vi "resonant.scan.engine.8or12kHz5ch_MD.vi"() -> ()   [LabVIEW 2012]
uses:
  <vilib>/Utility/VariantDataType/Type.ctl
  GFG/GFGbooleanGet.vi
  GFG/GFGnumericGet.vi
  GFG/GFGfpRefGet.vi
  <vilib>/Utility/error.llb/Error Cluster From Error Code.vi
  <vilib>/RVI Host/nirviSupport.llb/nirviErrorClusterFromErrorCode.vi
  <vilib>/rvi/errors/niLvFpgaAdjustHostInterfaceError.vi
  <vilib>/FPGAPlugInAG/PXIe-7962R/niLvFpga_Abort_PXIe-7962R.vi
  <vilib>/FPGAPlugInAG/PXIe-7962R/niLvFpga_Close_PXIe-7962R.vi
  <vilib>/rvi/interface/nirviMethod/nirviMethod.xnode
  FPGA/FPGA lvproj/FPGA Bitfiles/4chresonancescan_PXIe-7962R_5ch8or12kHzreson_D7lwWdudtb8.lvbitx
  <vilib>/rvi/interface/nirviCloseFPGA/nirviCloseFPGA.xnode
  GFG/GFG library.lvlib
  <vilib>/Utility/VariantDataType/VariantType.lvlib
  <vilib>/rvi/errors/niLvFpgaMergeErrorWithErrorCode.vi
  <vilib>/rvi/interface/nirviMethod/StockFPGA_InlinedMethodWaitForSingleIRQ.vi
  <vilib>/FPGAPlugInAG/PXIe-7962R/niLvFpga_WaitOnIrq_PXIe-7962R.vi
  <vilib>/FPGAPlugInAG/PXIe-7962R/niLvFpga_AcknowledgeIrq_PXIe-7962R.vi
  <vilib>/FPGAPlugInAG/PXIe-7962R/niLvFpga_ReadFifo_PXIe-7962R.vi
panel:
  out "x/y":dbl format="%#_6f"
  out "max Elements Remaining 2":u32
  out "Array":i16[][][](array[numeric])
  out "size(s)":i32[](array[numeric])
  out "Elements Remaining":u32
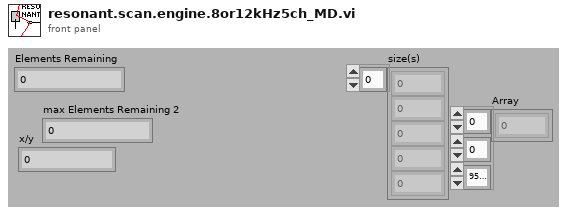
[diagram p1: front panel]
types:
  T1 = enum8{"Enabled", "Disabled", "Disabled and Grayed Out"}
  T2 = cluster{"WaveformChartRef":refnum<vi>, "DigitalRef":refnum<vi>, "ArrayRef":refnum<vi>, "TabControlRef":refnum<vi>, "EnumRef":refnum<vi>, "RingRef":refnum<vi>, "BooleanRef":refnum<vi>, "KnobRef":refnum<vi>, "SlideRef":refnum<vi>, "PathRef":refnum<vi>, "StringRef":refnum<vi>, "ComboBox":refnum<vi>, "WaveformGraphRef":refnum<vi>}
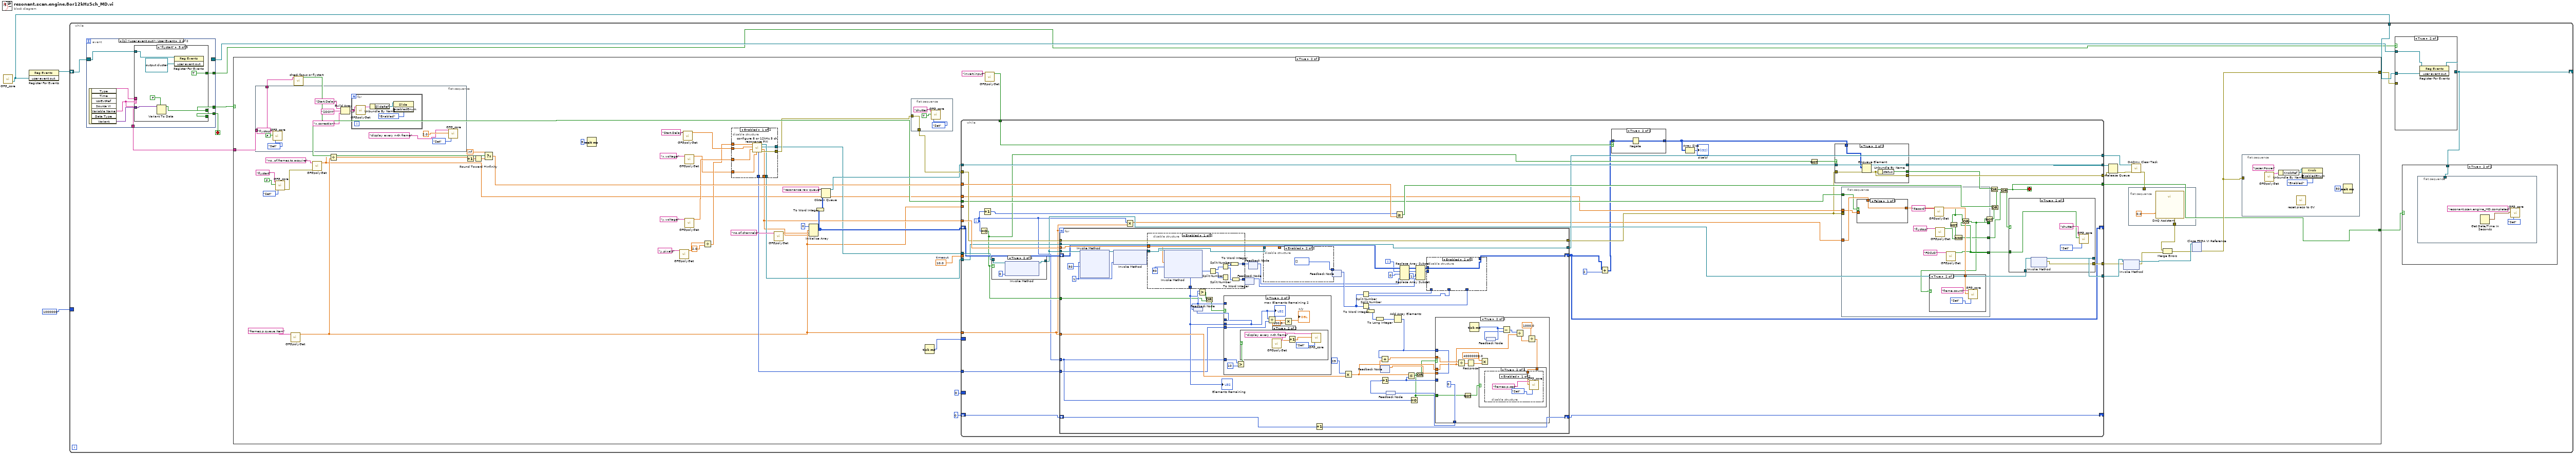
[diagram p0: block diagram]
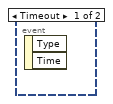
[diagram p4: hidden frame]
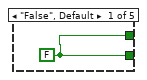
[diagram p5: hidden frame]
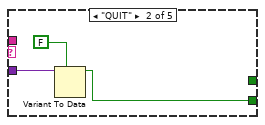
[diagram p6: hidden frame]
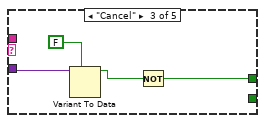
[diagram p7: hidden frame]
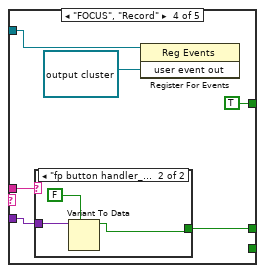
[diagram p8: hidden frame]
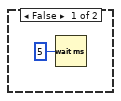
[diagram p10: hidden frame]
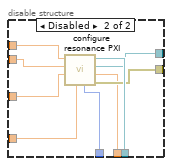
[diagram p11: hidden frame]
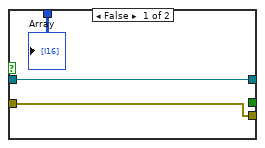
[diagram p12: hidden frame]
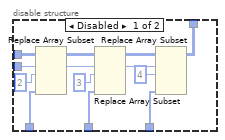
[diagram p13: hidden frame]
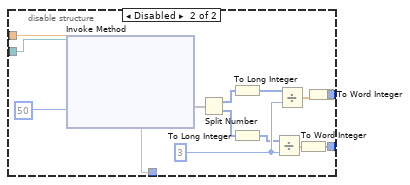
[diagram p14: hidden frame]
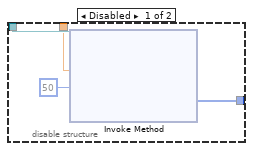
[diagram p15: hidden frame]
diagram:
  n1 = call "GFG_core.vi"() -> ("user event out"=w2:refnum<user-event>)  [unwired: 13 in, 6 out]
  n2 = register-events(w2) -> (reference out=w3:refnum<event-registration>)  [unwired: 2 in, 1 out]
  n3 = while {
    shift-right: [w4] -> _
    shift-left: w3 -> [w11]
    tunnel: w2 -> [w10]
    border: u32 1000000 ("Elements Remaining") -> [_]
    stop <- w12 stop-if-true
    n4 = event shown="[1] <user event out>: User Event" {
      selector: w11 -> [_ w24]
      dyn-events: [_ _] -> w8
      timeout: _ -> [_ _]
      tunnel: [_ w28] -> w13
      tunnel: [_ w27] -> w12
      tunnel: [_ w23] -> w7
      tunnel: [_ w22] -> w6
      event Timeout {
        n5 = event-data() -> ()  [unwired: 1 in, 2 out]
      }
      event User Event {
        n6 = event-data() -> ("Source VI"=w25:string, "Variable Name"=w22:string, "Variant"=w26:variant)  [unwired: 1 in, 4 out]
        n7 = case shown="\"flystart\"" w22 {
          tunnel: [w29 _ w33 w41 w46] -> w28
          tunnel: [w29 w30 _ _ _] -> w27
          tunnel: w26 -> [_ w32 w35 w42 w50]
          tunnel: w25 -> [_ _ _ w40 _]
          tunnel: w24 -> [_ _ _ w38 w47]
          tunnel: [_ _ _ TRUE TRUE] -> w23
          frame "False", Default {
            w29 = FALSE ("NewVal")
          }
          frame "QUIT" {
            n8 = Variant To Data(type=FALSE ("NewVal"), Variant=w32) -> (data=w30:bool)  [unwired: 1 in, 1 out]
          }
          frame "Cancel" {
            n9 = Variant To Data(type=FALSE ("NewVal"), Variant=w35) -> (data=w34:bool)  [unwired: 1 in, 1 out]
            n10 = Not(x=w34) -> (.not. x?=w33:bool)
          }
          frame "FOCUS", "Record" {
            n11 = case shown="\"fp button handler_MD.vi\"" w40 {
              tunnel: w42 -> [_ w44]
              tunnel: [_ w43] -> w41
              frame "False", Default {
              }
              frame "fp button handler_MD.vi" {
                n12 = Variant To Data(type=FALSE ("NewVal"), Variant=w44) -> (data=w43:bool)  [unwired: 1 in, 1 out]
              }
            }
            n13 = register-events(reference=w38, refnum<user-event> refnum ("user event out")) -> ()  [unwired: 1 in, 2 out]
          }
          frame "flystart" {
            n14 = Variant To Data(type=FALSE ("NewVal"), Variant=w50) -> (data=w46:bool)  [unwired: 1 in, 1 out]
            n15 = register-events(reference=w47, refnum<user-event> refnum ("user event out")) -> ()  [unwired: 1 in, 2 out]
          }
        }
      }
    }
    n16 = case shown="True" w13 {
      tunnel: [_ w88] -> w9
      tunnel: w6 -> [_ w56]
      tunnel: [_ w78] -> w5
      frame False {
        n17 = Wait (ms)(milliseconds to wait=u32 5) -> ()  [unwired: 1 out]
      }
      frame True {
        w109 = 10.0  # timeout
        n18 = flat-sequence {
          tunnel: w56 -> [w138]
          tunnel: [w138] -> w55
          frame #0 {
            n19 = call "GFG_core.vi"("Variable Name in"="flystop", "Variant in"=FALSE ("Boolean"), "Action"=enum16{"Init", "Set", "Get"}."Set") -> ()  [unwired: 10 in, 7 out]
            n20 = Build Array("Start.Delay" ("Variable Name in"), "ZOOM" ("Variable Name in"), "x.correction" ("Variable Name in")) -> (w133:string[])
            n21 = for {
              tunnel: w133 -> [w141] mode=indexing
              n22 = call-poly "GFGpolyGet.vi"("Variable Name in"=w141) -> ("output cluster"=w144:T2)  [unwired: 9 in, 1 out]
              n23 = Unbundle By Name(w144) -> ("SlideRef"=w142:refnum<vi>)
              n24 = property class="Slide"(reference=w142, "DisabledEnum"=T1."Enabled" ("Disabled")) -> ()  [unwired: 1 in, 2 out]
            }
            n25 = call "GFG_core.vi"("Variable Name in"="display every n-th frame" ("Tag in"), "Variant in"=2.0 ("Numeric"), "Action"=enum16{"Init", "Set", "Get"}."Set") -> ()  [unwired: 10 in, 7 out]
          }
        }
        n26 = call "GFG_core.vi"("Variable Name in"="flystart" ("Tag in"), "Variant in"=FALSE, "Action"=enum16{"Init", "Set", "Get"}."Set") -> ("error out"=w79:errorcluster)  [unwired: 10 in, 6 out]
        n27 = call-poly "GFGpolyGet.vi"("Variable Name in"="frames.p.queue.item" ("Tag in")) -> ("Numeric"=w61:dbl)  [unwired: 9 in, 1 out]
        n28 = call "check focus or flystart.vi"("x"=w55) -> ("x .or. y?"=w84:bool)  [unwired: 10 in]
        n29 = call-poly "GFGpolyGet.vi"("error in (no error)"=w79, "Variable Name in"="no..of.frames.to.acquire" ("Tag in")) -> ("Numeric"=w60:dbl)  [unwired: 8 in, 1 out]
        n30 = Divide(x=w60, y=w61) -> (x/y=w62:dbl)
        n31 = Increment(x=w62) -> (x+1=w57:dbl)
        n32 = Round Toward +Infinity(x=w57) -> (ceil(x): smallest int >= x=w59:dbl)
        n33 = Select(t=inf, s=w84, f=w59) -> (s? t:f=w85:dbl)
        n34 = Wait (ms)(milliseconds to wait=u32 5) -> ()  [unwired: 1 out]
        n35 = call-poly "GFGpolyGet.vi"("Variable Name in"="y.pixels" ("Tag in")) -> ("Numeric"=w103:dbl)  [unwired: 9 in, 1 out]
        n36 = call-poly "GFGpolyGet.vi"("Variable Name in"="Start.Delay" ("Tag in")) -> ("Numeric"=w75:dbl)  [unwired: 9 in, 1 out]
        n37 = call-poly "GFGpolyGet.vi"("Variable Name in"="x.voltage" ("Tag in")) -> ("Numeric"=w72:dbl)  [unwired: 9 in, 1 out]
        n38 = call-poly "GFGpolyGet.vi"("Variable Name in"="y.voltage" ("Tag in")) -> ("Numeric"=w74:dbl)  [unwired: 9 in, 1 out]
        n39 = Divide(x=w103, y=2.0 ("x")) -> (x/y=w73:dbl)
        n40 = disable-structure shown="Enabled" {
          disable-tunnel: w75 -> [w120 w123]
          disable-tunnel: w74 -> [w119 w125]
          disable-tunnel: w73 -> [w118 w122]
          disable-tunnel: w72 -> [w117 w124]
          disable-tunnel: [w116 w127] -> w71
          disable-tunnel: [w115 w129] -> w70
          disable-tunnel: [w114 w126] -> w66
          disable-tunnel: [w112 w128] -> w65
          disable-tunnel: [w113 w121] -> w63
          frame Enabled {
            n41 = call "configure 8 or 12kHz 5 ch resonance PXI.vi"("x resonant zoom voltage"=w117, "y-voltage"=w119, "Start Delay (Ticks)"=w120, "lines (2pi) per frame"=w118) -> ("error out"=w116:errorcluster, "pixels per frame"=w114:dbl, "FPGA VI Reference Out"=w112:refnum<k20>, "AO task out"=w115:refnum<k21>, "Actual Depth 3"=w113:u32)  [unwired: 3 in]
          }
          frame Disabled {
            n42 = call "configure resonance PXI.vi"("x resonant zoom voltage"=w124, "y-voltage"=w125, "Start Delay (Ticks)"=w123, "lines (2pi) per frame"=w122) -> ("error out"=w127:errorcluster, "pixels per frame"=w126:dbl, "FPGA VI Reference Out"=w128:refnum<k20>, "AO task out"=w129:refnum<k21>, "Actual Depth"=w121:u32)  [unwired: 3 in]
          }
        }
        n43 = call-poly "GFGpolyGet.vi"("Variable Name in"="no.of.channels" ("Tag in")) -> ("Numeric"=w69:dbl)  [unwired: 9 in, 1 out]
        n44 = Initialize Array(i16 0, w61, w69, w66) -> (w95:i16[][][])
        n45 = To Word Integer(number=w95) -> (16bit integer=w53:i16[][][])
        n46 = Obtain Queue(name (unnamed)="resonance raw queue", element data type=w53) -> (queue out=w96:refnum<queue>)  [unwired: 3 in, 2 out]
        n47 = flat-sequence {
          tunnel: [w152] -> w105
          tunnel: w71 -> [w152]
          frame #0 {
            n48 = call "GFG_core.vi"("Variable Name in"="shutter" ("Tag in"), "Variant in"=TRUE, "Action"=enum16{"Init", "Set", "Get"}."Set") -> ()  [unwired: 10 in, 7 out]
          }
        }
        n49 = Tick Count (ms)() -> (millisecond timer value=w54:u32)
        n50 = call-poly "GFGpolyGet.vi"("Variable Name in"="invert.input" ("Tag in")) -> ("Boolean"=w106:bool)  [unwired: 10 in]
        n51 = while {
          tunnel: w70 -> [w182]
          tunnel: [w181] -> w111
          tunnel: [w192] -> w68
          tunnel: w96 -> [w195]
          tunnel: [w194] -> w110
          tunnel: w85 -> [w193]
          tunnel: w109 -> [_]
          tunnel: w105 -> [w183]
          tunnel: w106 -> [w190]
          tunnel: w65 -> [w186]
          tunnel: w66 -> [w184]
          tunnel: [w180] -> w94
          tunnel: [w179] -> w92
          tunnel: w84 -> [w178]
          tunnel: w60 -> [w177]
          tunnel: [w172] -> w78
          shift-right: [w158] -> _
          shift-left: w95 -> [w185]
          tunnel: w61 -> [w164]
          tunnel: w61 -> [_]
          border: 0 ("x+y") -> [_]
          tunnel: w63 -> [w166]
          shift-right: [w161] -> _
          shift-left: 0 ("x+y") -> [w162]
          border: w54 -> [_]
          i -> [w160]
          stop <- w172 stop-if-true
          n52 = Equal To 0?(x=w160) -> (x = 0?=w167:bool)
          n53 = Increment(x=w160) -> (x+1=w163:i32)
          n54 = case shown="True" w167 {
            tunnel: w186 -> [w331 w334]
            tunnel: [w331 w333] -> w171
            frame False {
            }
            frame True {
              n55 = xnode "Invoke Method"("FPGA VI Reference In"=w334, "IRQ Number(s)"=0) -> ("FPGA VI Reference Out"=w333:refnum<k20>)  [unwired: 1 in, 1 out]
            }
          }
          n56 = for {
            N: w164 -> [_]
            tunnel: [w254] -> w168
            tunnel: w183 -> [w254]
            tunnel: w182 -> [w252]
            tunnel: w184 -> [w250]
            tunnel: w171 -> [w253]
            shift-right: [w244] -> w158
            shift-left: w185 -> [w248]
            tunnel: [w252] -> w181
            tunnel: w164 -> [w232]
            tunnel: w167 -> [w224]
            tunnel: w166 -> [w223]
            shift-right: [w221] -> w161
            shift-left: w162 -> [w222]
            tunnel: w160 -> [w214]
            i -> [w243]
            w220 = 1 ("IRQ Number(s)")
            n57 = xnode "Invoke Method"("FPGA VI Reference In"=w253, "IRQ Number(s)"=w220, "Timeout (ms)"=50) -> ("FPGA VI Reference Out"=w219:refnum<k20>)  [unwired: 1 in, 3 out]
            n58 = xnode "Invoke Method"("FPGA VI Reference In"=w219, "IRQ Number(s)"=w220) -> ("FPGA VI Reference Out"=w251:refnum<k20>)  [unwired: 1 in, 1 out]
            n59 = disable-structure shown="Enabled" {
              disable-tunnel: w251 -> [w277 w287]
              disable-tunnel: w250 -> [w276 w286]
              disable-tunnel: [w275 w280] -> w228
              disable-tunnel: [w268 w282] -> w208
              disable-tunnel: [w267 w281] -> w207
              frame Enabled {
                n60 = xnode "Invoke Method"("FPGA VI Reference In"=w277, "Number of Elements"=w276, "Timeout (ms)"=50) -> ("Data"=w273:u64[], "Elements Remaining"=w275:u32)  [unwired: 1 in, 2 out]
                n61 = Split Number(x=w273) -> (hi(x)=w272:u32[], lo(x)=w271:u32[])
                n62 = Split Number(x=w272) -> (hi(x)=w270:u16[], lo(x)=w269:u16[])
                n63 = Split Number(x=w271) -> ()  [unwired: 2 out]
                n64 = To Word Integer(number=w270) -> (16bit integer=w268:i16[])
                n65 = To Word Integer(number=w269) -> (16bit integer=w267:i16[])
              }
              frame Disabled {
                w284 = 3
                n66 = xnode "Invoke Method"("FPGA VI Reference In"=w287, "Number of Elements"=w286, "Timeout (ms)"=50) -> ("Data"=w291:void[], "Elements Remaining"=w280)  [unwired: 1 in, 2 out]
                n67 = Split Number(x=w291) -> (hi(x)=w289:u16[], lo(x)=w288:u16[])
                n68 = To Long Integer(number=w289) -> (32bit integer=w285:i32[])
                n69 = To Long Integer(number=w288) -> (32bit integer=w278:i32[])
                n70 = Divide(x=w278, y=w284) -> (x/y=w279:dbl[])
                n71 = Divide(x=w285, y=w284) -> (x/y=w283:dbl[])
                n72 = To Word Integer(number=w279) -> (16bit integer=w281:i16[])
                n73 = To Word Integer(number=w283) -> (16bit integer=w282:i16[])
              }
            }
            "Elements Remaining" <- w228
            n74 = feedback #1() -> (w226:u32)
            n75 = Greater?(x=w228, y=w226) -> (0:w229:bool)
            n76 = Or(x=w229, y=w224) -> (x .or. y?=w225:bool)
            n77 = case shown="True" w225 {
              tunnel: w228 -> [_ w305]
              tunnel: [w297 w305] -> w227
              tunnel: w226 -> [w297 _]
              tunnel: w223 -> [_ w304]
              tunnel: w214 -> [_ w300]
              frame False {
              }
              frame True {
                n78 = Greater?(x=w300, y=10) -> (0:w298:bool)
                n79 = case shown="True" w298 {
                  frame False {
                  }
                  frame True {
                    w308 = "display every n-th frame" ("Tag in")
                    n80 = call-poly "GFGpolyGet.vi"("Variable Name in"=w308) -> ("Numeric"=w307:dbl)  [unwired: 9 in, 1 out]
                    n81 = Increment(x=w307) -> (x+1=w306:dbl)
                    n82 = call "GFG_core.vi"("Variable Name in"=w308, "Variant in"=w306, "Action"=enum16{"Init", "Set", "Get"}."Set") -> ()  [unwired: 10 in, 7 out]
                  }
                }
                n83 = Divide(x=w305, y=w304) -> (x/y=w303:dbl)
                n84 = Multiply(x=w303, y=100.0) -> (x*y=→"x/y":dbl)
                "max Elements Remaining 2" <- w305
              }
            }
            n85 = feedback-in #1(w227) -> ()
            n86 = feedback-in #2(w207) -> ()
            n87 = feedback #2() -> (w206:i16[])  [unwired: 1 in]
            n88 = feedback-in #3(w208) -> ()
            n89 = feedback #3() -> (w205:i16[])  [unwired: 1 in]
            n90 = disable-structure shown="Enabled" {
              disable-tunnel: w251 -> [w294 _]
              disable-tunnel: w250 -> [w293 _]
              disable-tunnel: [w292 u32[] [] ("lo(x)")] -> w249
              frame Disabled {
                n91 = xnode "Invoke Method"("FPGA VI Reference In"=w294, "Number of Elements"=w293, "Timeout (ms)"=50) -> ("Data"=w292:u32[])  [unwired: 1 in, 3 out]
              }
              frame Enabled {
              }
            }
            n92 = Increment(x=w222) -> (x+1=w221:i32)
            n93 = feedback-in #4(w249) -> ()
            n94 = feedback #4() -> (w209:u32[])  [unwired: 1 in]
            n95 = Multiply(x=u32 25, y=w232) -> (x*y=w231:dbl)
            n96 = Split Number(x=w209) -> (hi(x)=w212:u16[], lo(x)=w211:u16[])
            n97 = Split Number(x=w209) -> (hi(x)=w210:u16[], lo(x)=w230:u16[])
            n98 = To Word Integer(number=w230) -> (16bit integer=w216:i16[])
            n99 = To Long Integer(number=w216) -> (32bit integer=w237:i32[])
            n100 = feedback #5() -> (w241:dbl)  [unwired: 1 in]
            n101 = feedback #6() -> (w236:i32)
            n102 = Increment(x=w236) -> (x+1=w239:i32)
            n103 = Add Array Elements(numeric array=w237) -> (sum=w217:i32)
            n104 = Add(x=w217, y=w241) -> (x+y=w235:dbl)
            n105 = Replace Array Subset(array=w248, new element=w205, index (dim 0)=w243, index (dim 1)=0 ("disabled index (row)")) -> (w246:i16[][][])  [unwired: 1 in]
            n106 = Less Or Equal?(x=w231, y=w239) -> (x <= y?=w238:bool)
            n107 = Equal To 0?(x=w214) -> (x = 0?=w213:bool)
            n108 = Or(x=w213, y=w238) -> (x .or. y?=w215:bool)
            n109 = Replace Array Subset(array=w246, new element=w206, index (dim 0)=w243, index (dim 1)=1 ("disabled index (col)")) -> (w245:i16[][][])  [unwired: 1 in]
            n110 = disable-structure shown="Enabled" {
              disable-tunnel: w245 -> [w265 w266]
              disable-tunnel: [w262 w266] -> w244
              disable-tunnel: w243 -> [w261 _]
              disable-tunnel: w212 -> [w257 _]
              disable-tunnel: w211 -> [w256 _]
              disable-tunnel: w210 -> [w255 _]
              frame Disabled {
                n111 = Replace Array Subset(array=w265, new element=w257, index (dim 0)=w261, index (dim 1)=2 ("disabled index (col)")) -> (w264:i16[][][])  [unwired: 1 in]
                n112 = Replace Array Subset(array=w264, new element=w256, index (dim 0)=w261, index (dim 1)=3 ("disabled index (col)")) -> (w263:i16[][][])  [unwired: 1 in]
                n113 = Replace Array Subset(array=w263, new element=w255, index (dim 0)=w261, index (dim 1)=4 ("disabled index (row)")) -> (w262:i16[][][])  [unwired: 1 in]
              }
              frame Enabled {
              }
            }
            n114 = case shown="True" w215 {
              tunnel: w239 -> [w311 _]
              tunnel: [w311 0 ("x+y")] -> w240
              tunnel: w217 -> [_ w321]
              tunnel: w231 -> [_ w317]
              tunnel: w235 -> [w310 w322]
              tunnel: [w310 w321] -> w234
              tunnel: w213 -> [_ w313]
              frame False {
              }
              frame True {
                n115 = Divide(x=w322, y=w317) -> (x/y=w325:dbl)
                n116 = Not(x=w313) -> (.not. x?=w312:bool)
                n117 = Reciprocal(x=w325) -> (1/x=w324:dbl)
                n118 = Tick Count (ms)() -> (millisecond timer value=w320:u32)
                n119 = Multiply(x=40000000.0, y=w324) -> ()  [unwired: 1 out]
                n120 = feedback #7() -> (w319:u32)
                n121 = feedback-in #7(w320) -> ()
                n122 = Subtract(x=w320, y=w319) -> (x-y=w318:u32)
                n123 = Divide(x=w318, y=w317) -> (x/y=w316:dbl)
                n124 = Divide(x=1000.0, y=w316) -> (x/y=w314:dbl)
                n125 = case shown="True" w312 {
                  tunnel: w314 -> [_ w327]
                  frame False {
                  }
                  frame True {
                    n126 = disable-structure shown="Enabled" {
                      disable-tunnel: w327 -> [w328 _]
                      frame Enabled {
                        n127 = call "GFG_core.vi"("Variable Name in"="frames.p.sec", "Variant in"=w328, "Action"=enum16{"Init", "Set", "Get"}."Set") -> ()  [unwired: 10 in, 7 out]
                      }
                      frame Disabled {
                      }
                    }
                  }
                }
              }
            }
            n128 = feedback-in #5(w234) -> ()
            n129 = feedback-in #6(w240) -> ()
          }
          n130 = Multiply(x=w160, y=w164) -> (x*y=w165:dbl)
          n131 = Greater Or Equal?(x=w163, y=w193) -> (x >= y?=w188:bool)
          n132 = Add(x=w158, y=i16 2 ("millisecond timer value")) -> (x+y=w156:i16[][][])
          n133 = case shown="True" w190 {
            tunnel: [w335 w337] -> w159
            tunnel: w156 -> [w335 w336]
            frame False {
            }
            frame True {
              n134 = Negate(x=w336) -> (-x=w337:i16[][][])
            }
          }
          n135 = Array Size(array=w159) -> (size(s)=→"size(s)":i32[])
          n136 = Not(x=w167) -> (.not. x?=w169:bool)
          n137 = case shown="True" w169 {
            tunnel: w159 -> [w196 w199]
            tunnel: w195 -> [w198 w204]
            tunnel: [w198 w203] -> w194
            tunnel: [w197 w202] -> w192
            tunnel: [_ w201] -> w189
            tunnel: w168 -> [w197 w200]
            frame False {
              "Array" <- w196
            }
            frame True {
              n138 = Enqueue Element(queue=w204, element=w199, error in (no error)=w200) -> (queue out=w203:refnum<queue>, error out=w202:errorcluster)  [unwired: 1 in, 1 out]
              n139 = Unbundle By Name(w202) -> ("status"=w201:bool)
            }
          }
          n140 = flat-sequence {
            tunnel: [w341] -> w175
            tunnel: w168 -> [_]
            tunnel: w165 -> [w348]
            tunnel: w178 -> [w346]
            tunnel: w177 -> [w345]
            tunnel: [w338] -> w174
            tunnel: [w339] -> w173
            frame #0 {
              n141 = case shown="False" w346 {
                tunnel: w345 -> [_ w357]
                tunnel: w348 -> [w354 w356]
                tunnel: [w354 w355] -> w347
                frame False {
                }
                frame True {
                  n142 = Quotient & Remainder(x=w356, y=w357) -> (x-y*floor(x/y)=w355:dbl)  [unwired: 1 out]
                }
              }
              n143 = call-poly "GFGpolyGet.vi"("Variable Name in"="Record") -> ("Boolean"=w342:bool)  [unwired: 10 in]
              n144 = call-poly "GFGpolyGet.vi"("Variable Name in"="flystop") -> ("Boolean"=w340:bool)  [unwired: 10 in]
              n145 = call-poly "GFGpolyGet.vi"("Variable Name in"="FOCUS") -> ("Boolean"=w341:bool)  [unwired: 10 in]
              n146 = Not(x=w342) -> (.not. x?=w343:bool)
              n147 = And(x=w343, y=w340) -> (x .and. y?=w339:bool)
              n148 = Or(x=w342, y=w341) -> (x .or. y?=w338:bool)
              n149 = case shown="True" w338 {
                tunnel: w347 -> [_ w351]
                frame False {
                }
                frame True {
                  n150 = call "GFG_core.vi"("Variable Name in"="frame.count", "Variant in"=w351, "Action"=enum16{"Init", "Set", "Get"}."Set") -> ()  [unwired: 10 in, 7 out]
                }
              }
            }
          }
          n151 = Not(x=w174) -> (.not. x?=w191:bool)
          n152 = Or(x=w188, y=w191) -> (x .or. y?=w187:bool)
          n153 = Or(x=w189, y=w187) -> (x .or. y?=w176:bool)
          n154 = Or(x=w176, y=w173) -> (x .or. y?=w172:bool)
          n155 = case shown="True" w172 {
            tunnel: w171 -> [w358 w362]
            tunnel: [w358 w361] -> w180
            tunnel: [_ w360] -> w179
            tunnel: w175 -> [_ w359]
            frame False {
            }
            frame True {
              n156 = xnode "Invoke Method"("FPGA VI Reference In"=w362) -> ("FPGA VI Reference Out"=w361:refnum<k20>, "error out"=w360:errorcluster)  [unwired: 1 in]
              n157 = call "GFG_core.vi"("Variable Name in"="shutter" ("Tag in"), "Variant in"=w359, "Action"=enum16{"Init", "Set", "Get"}."Set") -> ()  [unwired: 10 in, 7 out]
            }
          }
        }
        n158 = Release Queue(queue=w110, error in (no error)=w68) -> (error out=w108:errorcluster)  [unwired: 1 in, 2 out]
        n159 = xnode "Invoke Method"("FPGA VI Reference In"=w94, "error in"=w92) -> ("FPGA VI Reference Out"=w93:refnum<k20>, "error out"=w91:errorcluster)
        n160 = flat-sequence {
          tunnel: [w145] -> w90
          tunnel: w67 -> [_]
          frame #0 {
            n161 = call "DAQ Assistant"("data"=0.0) -> ("error out"=w145:errorcluster)  [unwired: 17 in, 1 out]
          }
        }
        n162 = call <vilib>:"DAQmx Clear Task.vi"("task in"=w111, "error in"=w108) -> ("error out"=w67:errorcluster)  [unwired: 13 in]
        n163 = Merge Errors(w90, w91) -> (w89:errorcluster)
        n164 = xnode "Close FPGA VI Reference"("FPGA VI Reference In"=w93, "error in"=w89) -> ("error out"=w88:errorcluster)
        n165 = flat-sequence {
          tunnel: w88 -> [_]
          frame #0 {
            n166 = call-poly "GFGpolyGet.vi"("Variable Name in"="Laser.Power") -> ("output cluster"=w151:T2)  [unwired: 9 in, 1 out]
            n167 = Unbundle By Name(w151) -> ("KnobRef"=w148:refnum<vi>)
            n168 = call "reset piezo to 0V.vi"() -> ()  [unwired: 11 in, 1 out]
            n169 = property class="Knob"(reference=w148, "DisabledEnum"=T1."Enabled" ("Disabled")) -> ()  [unwired: 1 in, 2 out]
            n170 = Wait (ms)(milliseconds to wait=u32 50) -> ()  [unwired: 1 out]
          }
        }
      }
    }
    n171 = case shown="True" w7 {
      tunnel: w10 -> [_ w21]
      tunnel: w9 -> [_ _]
      tunnel: [w18 w20] -> w4
      tunnel: w8 -> [w18 w19]
      frame False {
      }
      frame True {
        n172 = register-events(reference=w19, w21) -> (reference out=w20:refnum<event-registration>)  [unwired: 1 in, 1 out]
      }
    }
    n173 = case shown="True" w5 {
      tunnel: w4 -> [_ w14]
      frame False {
      }
      frame True {
        n174 = flat-sequence {
          tunnel: w14 -> [_]
          frame #0 {
            n175 = Get Date/Time In Seconds() -> (seconds since 1Jan1904=w15:timestamp)
            n176 = call "GFG_core.vi"("Variable Name in"="resonant.scan.engine_MD.completed", "Variant in"=w15, "Action"=enum16{"Init", "Set", "Get"}."Set") -> ()  [unwired: 10 in, 7 out]
          }
        }
      }
    }
  }
